vi "Cleanup.vi"(8 "error in":errorcluster, 11 "PCAP Frame Logger in":refnum<class "PCAP Frame Logger.lvclass">) -> (0 "error out":errorcluster, 3 "PCAP Frame Logger out":refnum<class "PCAP Frame Logger.lvclass">)   [LabVIEW 2020, in "Frame Logging.lvlib" / "PCAP Frame Logger.lvclass"]
uses:
  PCAP Frame Logger.lvclass
  PCAP Frame Logger.lvclass/PCAP Frame Logger.ctl
  <vilib>/nisyscfg/Close (System).vi
  libpcaplv/libpcaplv.lvlib
  <vilib>/nisyscfg/nisyscfg.lvlib
  <vilib>/Utility/SystemLogging/NI_SystemLogging.lvlib
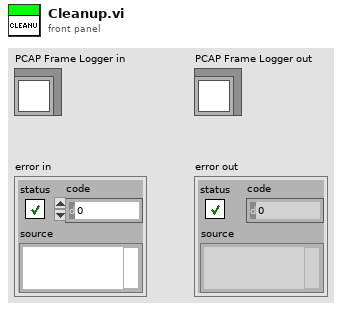
[diagram p1: front panel]
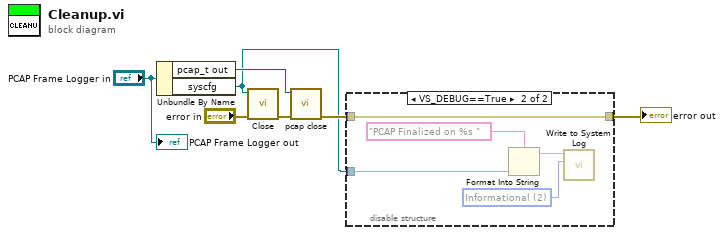
[diagram p0: block diagram]
diagram:
  n1 = Unbundle By Name("PCAP Frame Logger in") -> ("pcap_t out"=w7:u64, "syscfg"=w1:refnum<k21>)
  n2 = call-poly <vilib>:"Close.vi"("error in (no error)"="error in", "Session in"=w1) -> ("error out"=w4:errorcluster)  [unwired: 9 in]
  n3 = call "pcap close.vi"("error in"=w4, "pcap_t in"=w7) -> ("error out"=w3:errorcluster)  [unwired: 9 in]
  n4 = disable-structure shown="VS_DEBUG==True" {
    disable-tunnel: w3 -> [_ w9]
    disable-tunnel: [_ w9] -> w2
    disable-tunnel: w1 -> [_ w8]
    frame condition #0 (active) {
    }
    frame condition #1 {
      w10 = 2 items=["Error", "Warning", "Informational"] ("severity")
      n5 = Format Into String(format string="PCAP Finalized on %s ", w8) -> (resulting string=w11:string)  [unwired: 2 in, 1 out]
      n6 = call <vilib>:"Write to System Log.vi"("severity"=w10, "message"=w11) -> ()  [unwired: 9 in, 1 out]
    }
  }
  "error out" <- w2
  "PCAP Frame Logger out" <- "PCAP Frame Logger in"
